vi "Check for Empty Response.vi"(8 "Error In":errorcluster, 11 "Response Format in":string) -> (0 "Error Out":errorcluster, 3 "Response Format out":string)   [LabVIEW 2018, in "Instrument Addon Scripting API.lvlib"]
uses:
  Instrument Addon Scripting API.lvlib
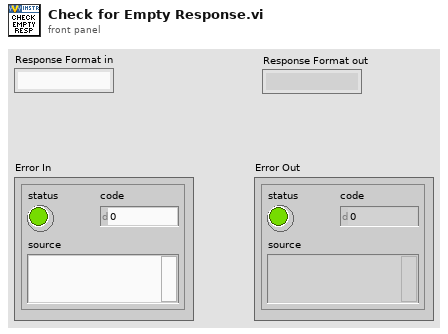
[diagram p1: front panel]
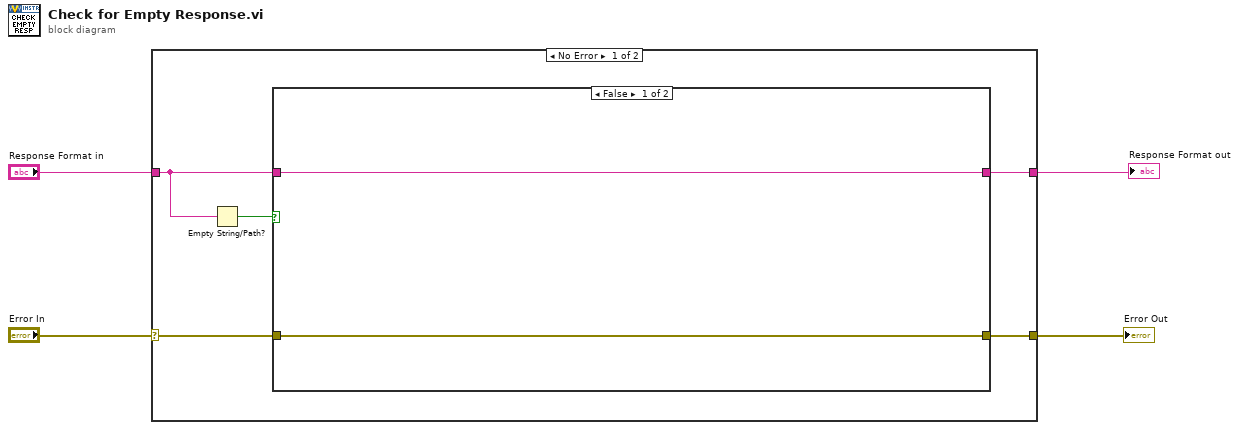
[diagram p0: block diagram]
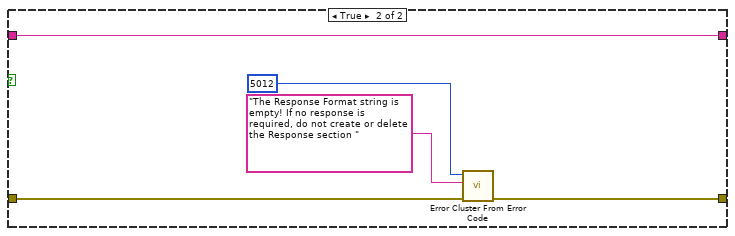
[diagram p2: hidden frame]
diagram:
  n1 = case shown="No Error" "Error In" {
    selector: "Error In" -> [w6 w17]
    tunnel: "Response Format in" -> [w8 w18]
    tunnel: [w7 w18] -> w3
    tunnel: [w5 w17] -> w1
    frame No Error {
      n2 = Empty String/Path?(string/path=w8) -> (empty?=w9:bool)
      n3 = case shown="False" w9 {
        tunnel: w8 -> [w11 w14]
        tunnel: [w11 w14] -> w7
        tunnel: w6 -> [w10 w13]
        tunnel: [w10 w12] -> w5
        frame False {
        }
        frame True {
          n4 = call <vilib>:"Error Cluster From Error Code.vi"("error in (no error)"=w13, "error message (\"\")"="The Response Format string is empty! If no response is required, do not create or delete the Response section " ("error message (\"\")"), "error code (0)"=5012) -> ("error out"=w12:errorcluster)  [unwired: 6 in]
        }
      }
    }
    frame Error {
    }
  }
  "Response Format out" <- w3
  "Error Out" <- w1
